vi "ULx Waveform Buffer Generation.vi"(4 "Offset":dbl format="%0.2p", 5 "Amplitude":dbl=2.0 format="%0.2p", 6 "Cycles per Buffer":dbl=1.0 format="%.2f", 7 "Samples per Buffer":dbl=1000.0, 8 "error in (no error)":errorcluster, 9 "Waveform Type":T1(ring), 10 "Max. Sample Clock Rate":dbl caption="Desired Sample Clock Rate" format="%.2f", 11 "Frequency":dbl=1000.0 caption="Desired Frequency" format="%.2f") -> (0 "error out":errorcluster, 1 "Sample Clock Rate":dbl caption="Desired Sample Clock Rate" format="%.2f", 3 "Waveform":waveform(dbl))   [LabVIEW 2015]
doc: "This subVI is used to create a Sine, Square, Triangle or Sawtooth Waveform. The inputs to this VI are the Waveform Type, which determines if the output waveform is a Sine, Square, Triangle, or Sawtooth Waveform, the amplitude, Desired Frequency, Samples per Buffer, and Cycles per Buffer. \n\nThe Desired Frequency, Samples per Buffer, and Cycles per Buffer are used to calculate the sample clock rate. The DAQmx Timing property node sets the sample clock rate for the device specified in the task/channels in control. \n\nThe actual, coerced, sample clock rate is returned and used as an input to the Basic Function Generator.vi. The Basic Function Generator returns a waveform of data with timing information.\n\nThe formula below was used to determine the sample clock rate:\n\nDesired Frequency=[(Cycles/Buffer)X(Sample Clock Rate)]/Samples per Buffer\n\nNote: The Block Diagram rearranges the variables to solve for Sample Clock Rate"
uses:
  <vilib>/measure/NI_MABase.lvlib
panel:
  out "Samples/cycle":dbl format="%0.2f"
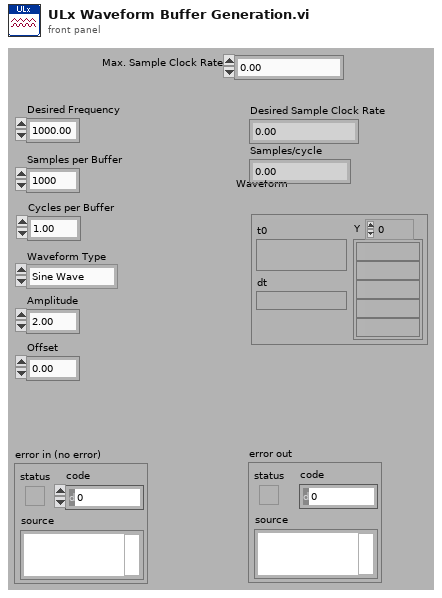
[diagram p1: front panel]
types:
  T1 = enum16{"Sine Wave", "Triangle Wave", "Square Wave", "Sawtooth Wave"}
  T2 = cluster{"Max. Sample Clock Rate":dbl, "Samples per Buffer":dbl}
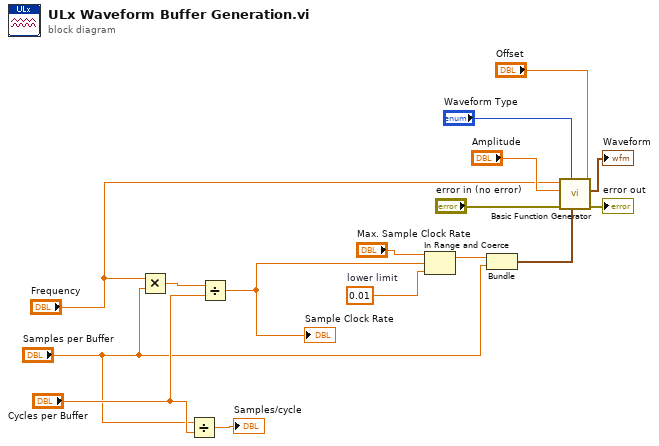
[diagram p0: block diagram]
diagram:
  w1 = 0.01  # lower limit
  n1 = Multiply(x="Frequency", y="Samples per Buffer") -> (x*y=w14:dbl)
  n2 = Divide(x="Samples per Buffer", y="Cycles per Buffer") -> (x/y=→"Samples/cycle":dbl)
  n3 = Divide(x=w14, y="Cycles per Buffer") -> (x/y=w4:dbl)
  "Sample Clock Rate" <- w4
  n4 = In Range and Coerce(upper limit="Max. Sample Clock Rate", x=w4, lower limit=w1) -> (coerced(x)=w2:dbl)  [unwired: 1 out]
  n5 = Bundle("Max. Sample Clock Rate"=w2, "Samples per Buffer"="Samples per Buffer") -> (w16:T2)  [unwired: 1 in]
  n6 = call <vilib>:"Basic Function Generator.vi"("offset"="Offset", "sampling info"=w16, "signal type"="Waveform Type", "error in (no error)"="error in (no error)", "amplitude"="Amplitude", "frequency"="Frequency") -> ("error out"=→"error out":errorcluster, "signal out"=→"Waveform":waveform(dbl))  [unwired: 3 in, 1 out]
